vi "Untitled 1.vi"() -> ()   [LabVIEW 2016]
uses:
  <vilib>/Instr/_visa.llb/VISA Configure Serial Port (Instr).vi
panel:
  in  "Calibration":u16(ring)=128 format="0x%x" items=["Set Photodiode Threshold"=128, "Get All Photodiode Thresholds"=129, "Set Photodiode Trimpot Setpoint"=130, "Get All Photodiode Trimpot Setpoints"=131, "Set Preamp Pump Current Setpoint"=132, "Get All Preamp Pump Current Setpoints"=133, "Set Temperature Sensor Warning Threshold"=134, "Get Temperature Sensor Warning Threshold"=135, "Set Temperature Sensor Fault Threshold"=136, "Get Temperature Sensor Fault Threshold"=137, "Set HPE Photodiode Auto Threshold Delay"=138, "Get HPE Photodiode Auto Threshold Delay"=139]
  in  "Extended Operation":u16(ring)=67 format="0x%x" items=["Set HPE Photodiode Signal Drop Tolerance"=67, "Get HPE Photodiode Signal Drop Tolerance"=68, "Switch HPE Photodiode Fault Enable"=69, "Get Temperature Sensor Status"=70, "Switch Communication Timeout Enable"=71]
  in  "Logistics":u16(ring)=65 format="0x%x" items=["Set RS-485 Address"=65, "Get RS-485 Address"=66]
  in  "Common Operation":u16(ring)=4 format="0x%d" items=["Undefined", "Query: Get Unit Information", "Cmd: Emission On", "Cmd: Emission Off", "Query: Get Basic Status", "Query: Get Core Status", "Query: Get Extended Status", "Cmd: Clear Faults", "Cmd: Set Power Mode"]
  out "error out":errorcluster
  in  "error in (no error)":errorcluster
  in  "baud rate (9600)":u32=115200
  in  "VISA resource name":refnum<visa-resource-name>
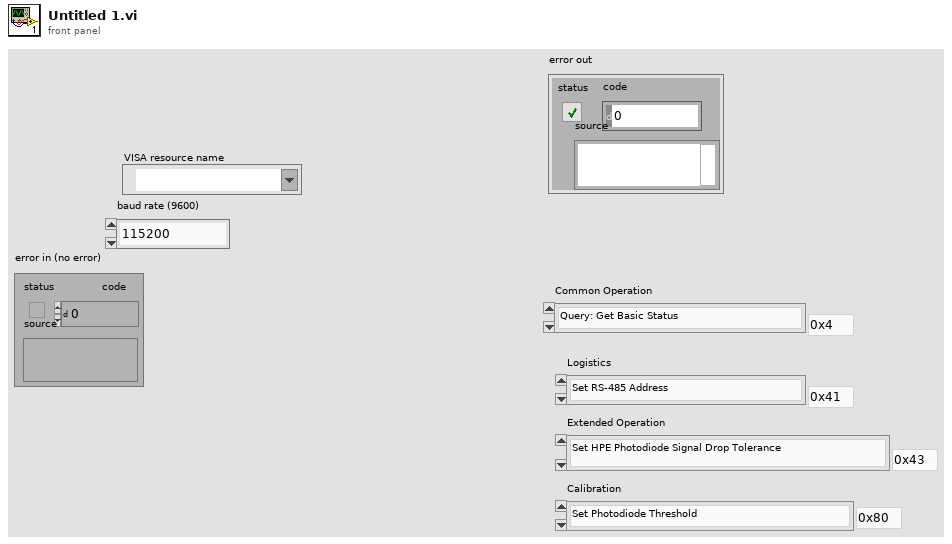
[diagram p1: front panel]
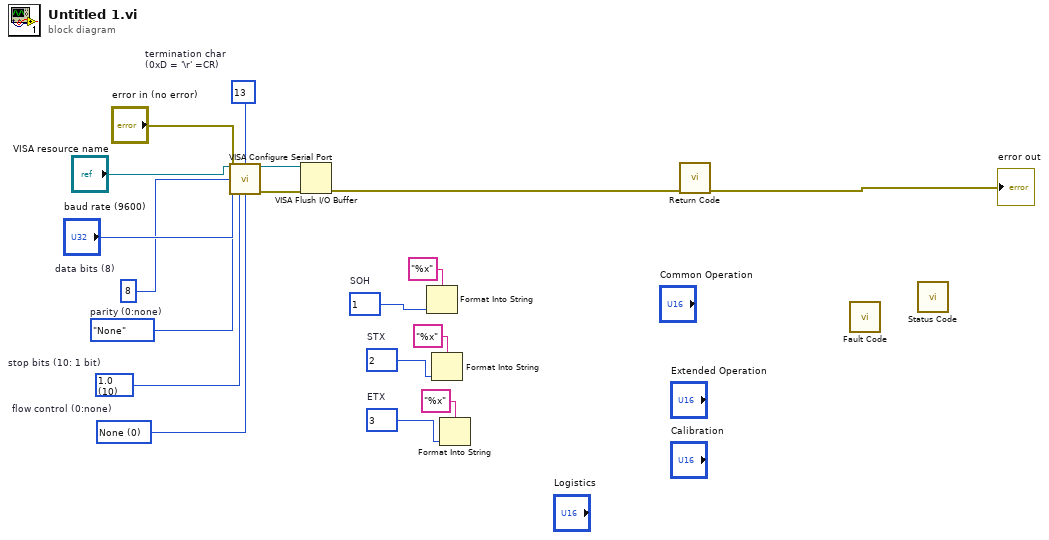
[diagram p0: block diagram]
diagram:
  w1 = u8 13  # termination char (0xD = '\r' =CR)
  w5 = 3  # ETX
  w4 = 2  # STX
  w9 = 1  # SOH
  w13 = u16 0 items=["None", "XON/XOFF", "RTS/CTS", "XON/XOFF & RTS/CTS", "DTR/DSR", "XON/XOFF & DTR/DSR"]  # flow control (0:none)
  w14 = u16 10 items=["1.0"=10, "1.5"=15, "2.0"=20]  # stop bits (10: 1 bit)
  w15 = enum16{"None", "Odd", "Even", "Mark", "Space"}."None"  # parity (0:none)
  w16 = u16 8  # data bits (8)
  n1 = call-poly "VISA Configure Serial Port"("VISA resource name"="VISA resource name", "termination char\n(0xA = '\\n' = LF)"=w1, "baud rate (9600)"="baud rate (9600)", "data bits (8)"=w16, "parity (0:none)"=w15, "error in (no error)"="error in (no error)", "stop bits (10: 1 bit)"=w14, "flow control (0:none)"=w13) -> ("VISA resource name out"=w10:refnum<visa-resource-name>, "error out"=w11:errorcluster)  [unwired: 6 in]
  n2 = VISA Flush I/O Buffer(VISA resource name=w10, error in (no error)=w11) -> (error out=w3:errorcluster)  [unwired: 1 in, 1 out]
  n3 = Format Into String(format string="%x", w9) -> ()  [unwired: 2 in, 2 out]
  n4 = Format Into String(format string="%x", w4) -> ()  [unwired: 2 in, 2 out]
  n5 = Format Into String(format string="%x", w5) -> ()  [unwired: 2 in, 2 out]
  n6 = call "Return Code.vi"("error in (no error)"=w3) -> ("error out"=→"error out":errorcluster)  [unwired: 9 in, 1 out]
  n7 = call "Fault Code.vi"() -> ()  [unwired: 10 in, 2 out]
  n8 = call "Status Code.vi"() -> ()  [unwired: 10 in, 2 out]
